vi "Read Multiple Measurements.vi"   [LabVIEW 2019, in "Agilent 681x Series.lvlib"]
doc: "Initiates and reads current or voltage measurement data.\n\n<B>Note:</B>\n\nThis VI changes the <B>Trigger Source</B> to <B>Bus</B> and uses a software trigger after the instrument is initiated. If you want to control the triggering and other features, please use the low level VIs."
uses:
  <instrlib>/Agilent 681x Series/Agilent 681x Series.lvlib
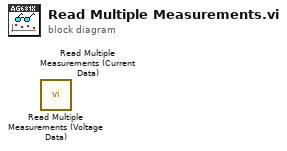
[diagram p0: block diagram]
diagram:
  n1 = call <instrlib>:"Read Multiple Measurements (Voltage Data).vi"() -> ()  [unwired: 11 in, 5 out]
  n2 = call <instrlib>:"Read Multiple Measurements (Current Data).vi"() -> ()  [unwired: 11 in, 5 out]
